vi "TEST.vi"() -> (8 "error out":errorcluster)   [LabVIEW 2021]
uses:
  Program Files (x86)/National Instruments/LabVIEW 2021/examples/Connectivity/Python/support/PythonVersionsEnum.ctl
panel:
  in  "Boolean":bool
  out "error out 2":errorcluster
  in  "error in (no error) 2":errorcluster
  out "Numeric 2":i32
  in  "stop":bool
  in  "error in (no error)":errorcluster
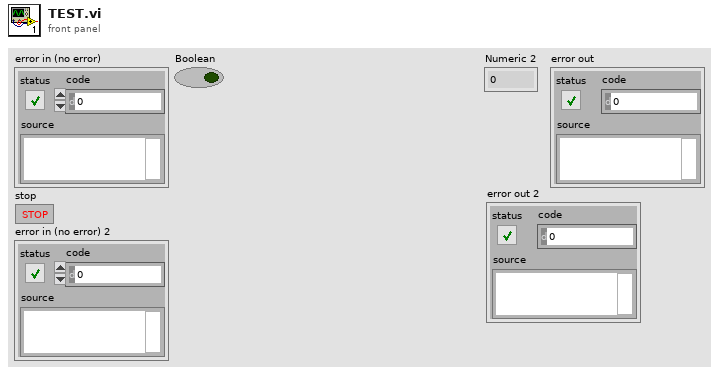
[diagram p1: front panel]
types:
  T1 = typedef "PythonVersionsEnum.ctl" = enum16{"3.6", "3.7", "3.8", "3.9"}
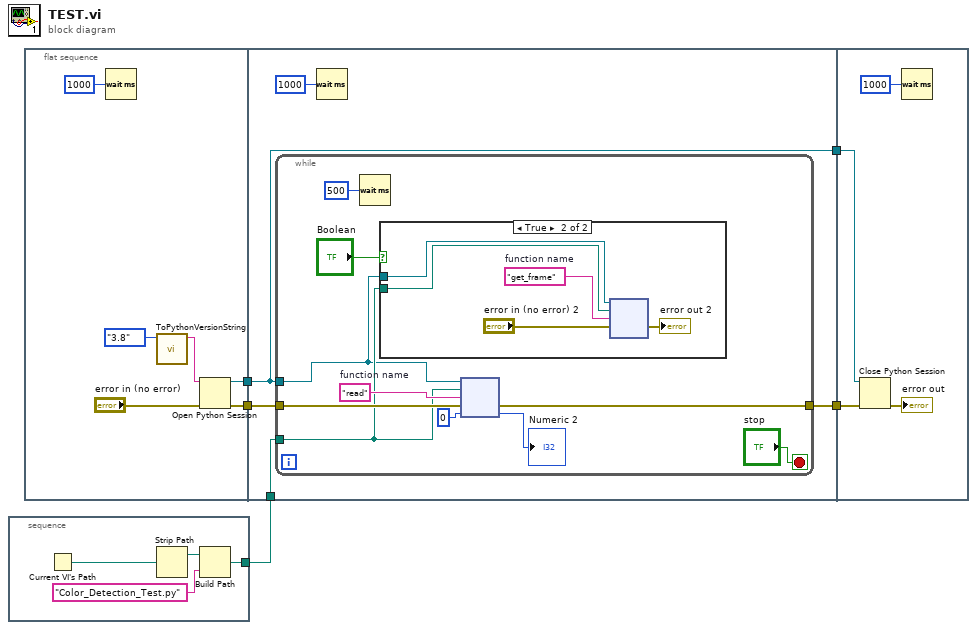
[diagram p0: block diagram]
diagram:
  n1 = stacked-sequence {
    tunnel: [w9] -> w5
    frame #0 {
      n2 = Current VI's Path() -> (path=w6:path)
      n3 = Strip Path(path=w6) -> (stripped path=w7:path)  [unwired: 1 out]
      n4 = Build Path(base path=w7, name or relative path="Color_Detection_Test.py") -> (appended path=w9:path)
    }
  }
  n5 = flat-sequence {
    tunnel: [w12] -> w4
    tunnel: [w11] -> w3
    tunnel: [w16] -> w2
    tunnel: [w19] -> w1
    tunnel: w3 -> [w16]
    tunnel: w4 -> [w17]
    tunnel: w5 -> [w20]
    tunnel: w2 -> [w37]
    tunnel: w1 -> [w36]
    frame #0 {
      n6 = Wait (ms)(milliseconds to wait=u32 1000) -> ()  [unwired: 1 out]
      n7 = call "ToPythonVersionString.vi"("python version"=PythonVersionsEnum."3.8") -> ("python version string"=w15:string)  [unwired: 10 in]
      n8 = Open Python Session(python version=w15, 3:"error in (no error)") -> (session out=w11:refnum<k35>, error out=w12:errorcluster)  [unwired: 1 in]
    }
    frame #1 {
      n9 = while {
        tunnel: [w25] -> w19
        tunnel: w17 -> [w24]
        tunnel: w20 -> [w23]
        tunnel: w16 -> [w21]
        stop <- "stop" stop-if-true
        w28 = "read"  # function name
        n10 = Wait (ms)(milliseconds to wait=u32 500) -> ()  [unwired: 1 out]
        n11 = case shown="True" "Boolean" {
          tunnel: w23 -> [_ w35]
          tunnel: w21 -> [_ w31]
          frame False {
          }
          frame True {
            w34 = "get_frame"  # function name
            n12 = node(w31, w35, w34, "error in (no error) 2") -> (→"error out 2":errorcluster)  [unwired: 2 in, 3 out]
          }
        }
        n13 = node(w21, w23, w28, w24, 0) -> (w25:errorcluster, →"Numeric 2":i32)  [unwired: 3 out]
      }
      n14 = Wait (ms)(milliseconds to wait=u32 1000) -> ()  [unwired: 1 out]
    }
    frame #2 {
      n15 = Close Python Session(session in=w37, error in=w36) -> (11:→"error out":errorcluster)
      n16 = Wait (ms)(milliseconds to wait=u32 1000) -> ()  [unwired: 1 out]
    }
  }
